vi "test_Multiple Local Enumerated Channel Command-Response Messages using Trigger with Padding and Protection.vi"(8 "error in (no error)":errorcluster, 11 "TestCase in":refnum<class "Common System Tests.lvclass">) -> (0 "error out":errorcluster, 3 "TestCase out":refnum<class "Common System Tests.lvclass">)   [LabVIEW 2018, in "Common System Tests.lvclass"]
uses:
  Common System Tests.lvclass
  C:/Dev/niveristand-custom-device-testing-tools/VeriStandTestCase/VeriStandTestCase.lvclass
  <vilib>/NI Veristand/Execution/Workspace/NI VeriStand - Set Multiple Channel Values.vi
  <vilib>/NI Veristand/Execution/Workspace/NI VeriStand - Get Multiple Channel Values.vi
  <vilib>/addons/_JKI Toolkits/VI Tester/TestCase.llb/TestCase.lvclass
  <vilib>/NI Veristand/Execution/Workspace/NI_VS Workspace ExecutionAPI.lvlib
  C:/Program Files (x86)/National Instruments/LabVIEW 2018/vi.lib/addons/_JKI Toolkits/VI Tester/TestCase.llb/TestCase.lvclass
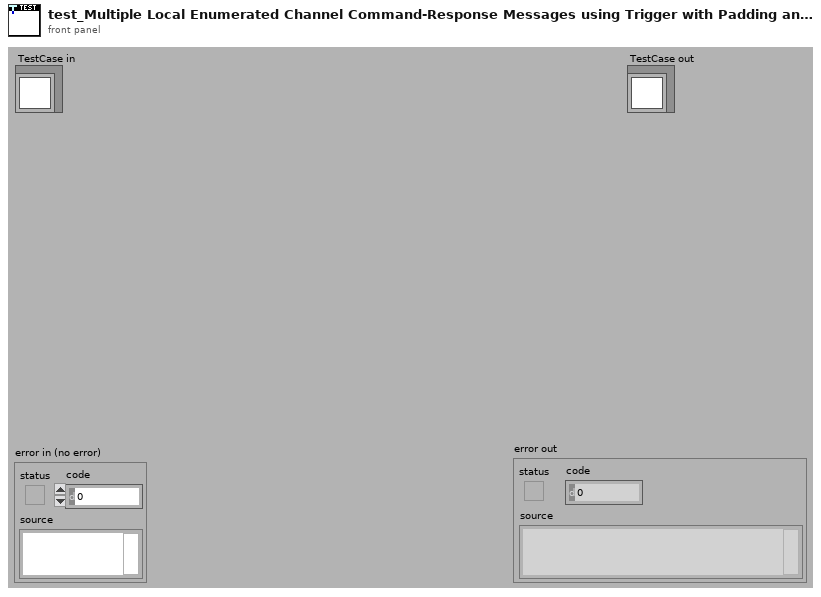
[diagram p1: front panel]
types:
  T1 = typedef "NI_VS Workspace ExecutionAPI.lvlib/WorkspaceAPI.ctl" = refnum<k24>
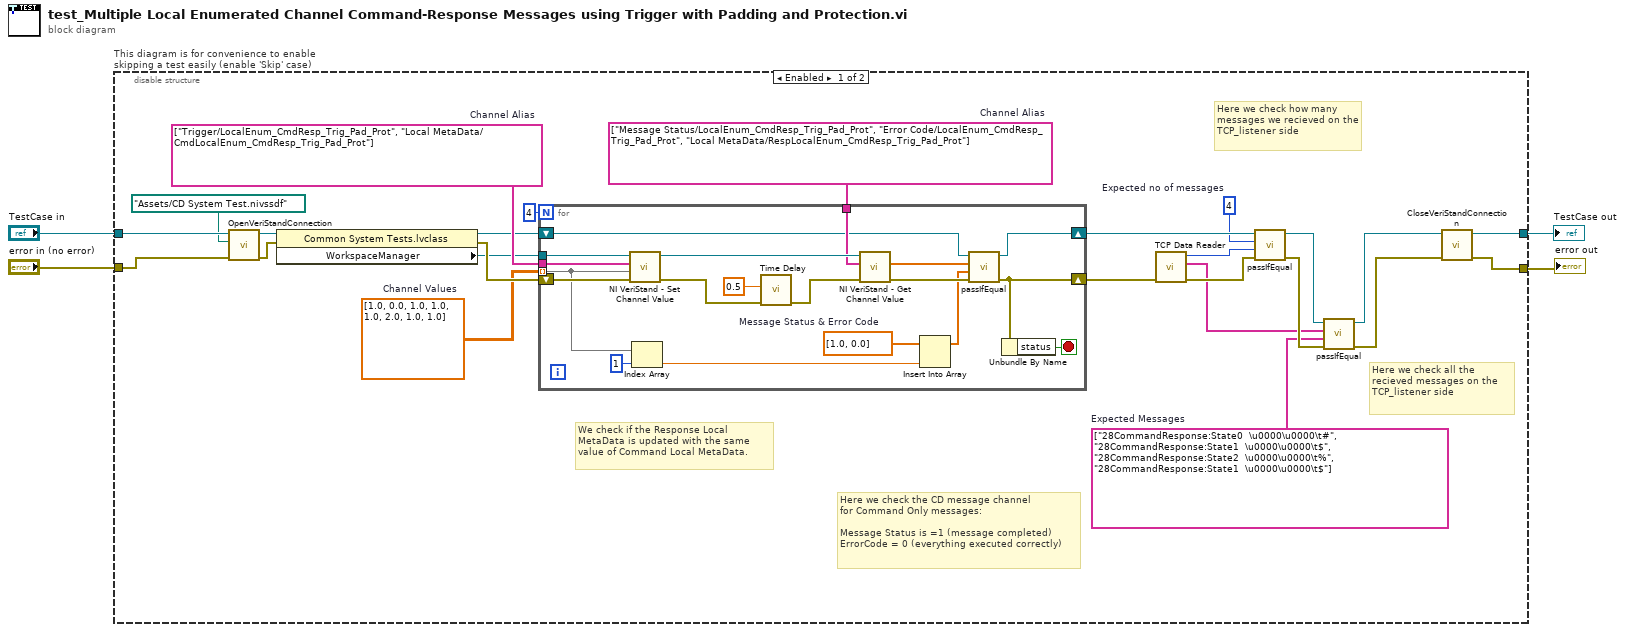
[diagram p0: block diagram]
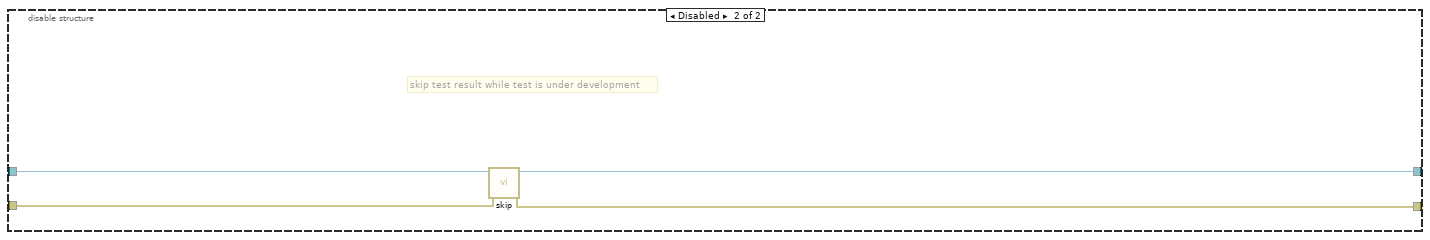
[diagram p2: hidden frame]
diagram:
  n1 = disable-structure "This diagram is for convenience to enable skipping a test easily (enable 'Skip' case)" shown="Enabled" {
    disable-tunnel: "TestCase in" -> [w27 w52]
    disable-tunnel: [w28 w50] -> w1
    disable-tunnel: [w29 w51] -> w3
    disable-tunnel: "error in (no error)" -> [w25 w49]
    frame Enabled {
      w5 = string[] ["28CommandResponse:State0  \u0000\u0000\t#", "28CommandResponse:State1  \u0000\u0000\t$", "28CommandResponse:State2  \u0000\u0000\t%", "28CommandResponse:State1  \u0000\u0000\t$"]  # Expected Messages
      w8 = 4  # Expected no of messages
      w17 = string[] ["Message Status/LocalEnum_CmdResp_Trig_Pad_Prot", "Error Code/LocalEnum_CmdResp_Trig_Pad_Prot", "Local MetaData/RespLocalEnum_CmdResp_Trig_Pad_Prot"]  # Channel Alias
      w20 = dbl[][] [[1.0, 0.0], [1.0, 1.0], [1.0, 2.0], [1.0, 1.0]]  # Channel Values
      w21 = string[] ["Trigger/LocalEnum_CmdResp_Trig_Pad_Prot", "Local MetaData/CmdLocalEnum_CmdResp_Trig_Pad_Prot"]  # Channel Alias
      # "We check if the Response Local MetaData is updated with the same value of Command Local MetaData."
      # "Here we check how many messages we recieved on the TCP_listener side"
      # "Here we check all the recieved messages on the TCP_listener side"
      # "Here we check the CD message channel\nfor Command Only messages:\n\nMessage Status is =1 (message completed)\nErrorCode = 0 (everything executed correctly)"
      n2 = call-dynamic "OpenVeriStandConnection.vi"("error in (no error)"=w25, "System Definition File"=path "Assets/CD System Test.nivssdf", "VeriStand Test Case in"=w27) -> ("error out"=w24:errorcluster, "VeriStand Test Case out"=w26:refnum<class "Common System Tests.lvclass">)  [unwired: 6 in, 1 out]
      n3 = property class="Common System Tests.lvclass"(reference=w26, error in=w24) -> (reference out=w18:refnum<class "Common System Tests.lvclass">, error out=w22:errorcluster, "WorkspaceManager"=w16:T1)
      n4 = for {
        N: 4 -> [_]
        tunnel: w16 -> [w48]
        tunnel: w21 -> [w46]
        tunnel: w20 -> [w33] mode=indexing
        shift-right: [w35] -> w7
        shift-left: w22 -> [w47]
        tunnel: w17 -> [w44]
        shift-right: [w39] -> w15
        shift-left: w18 -> [w40]
        stop <- w34 stop-if-true
        w36 = dbl[] [1.0, 0.0]  # Message Status & Error Code
        n5 = call-poly <vilib>:"NI VeriStand - Set Channel Value.vi"("error in (no error)"=w47, "Values"=w33, "Channels"=w46, "WorkspaceManager in"=w48) -> ("error out"=w42:errorcluster, "WorkspaceManager out"=w45:T1)  [unwired: 6 in]
        n6 = Index Array(array=w33, index=1) -> (element=w30:dbl)
        n7 = call "Time Delay"("error in (no error)"=w42, "Delay Time (s)"=0.5) -> ("error out"=w41:errorcluster)  [unwired: 9 in]
        n8 = call-poly <vilib>:"NI VeriStand - Get Channel Value.vi"("error in (no error)"=w41, "Channels"=w44, "WorkspaceManager in"=w45) -> ("error out"=w38:errorcluster, "Values"=w37:dbl[])  [unwired: 6 in, 1 out]
        n9 = Insert Into Array(array=w36, new element=w30) -> (w32:dbl[])  [unwired: 1 in]
        n10 = call-dynamic "passIfEqual.vi"("error in (no error)"=w38, "y"=w32, "x"=w37, "TestCase in"=w40) -> ("error out"=w35:errorcluster, "TestCase out"=w39:refnum<class "Common System Tests.lvclass">)  [unwired: 6 in]
        n11 = Unbundle By Name(w35) -> ("status"=w34:bool)
      }
      n12 = call "TCP Data Reader.vi"("error in (no error)"=w7) -> ("error out"=w13:errorcluster, "Recieved Messages"=w6:string[], "No of messages"=w9:i32)  [unwired: 8 in]
      n13 = call-dynamic "passIfEqual.vi"("error in (no error)"=w13, "y"=w9, "x"=w8, "TestCase in"=w15) -> ("error out"=w11:errorcluster, "TestCase out"=w14:refnum<class "Common System Tests.lvclass">)  [unwired: 6 in]
      n14 = call-dynamic "passIfEqual.vi"("error in (no error)"=w11, "y"=w5, "x"=w6, "TestCase in"=w14) -> ("error out"=w10:errorcluster, "TestCase out"=w12:refnum<class "Common System Tests.lvclass">)  [unwired: 6 in]
      n15 = call-dynamic "CloseVeriStandConnection.vi"("error in (no error)"=w10, "VeriStand Test Case in"=w12) -> ("error out"=w29:errorcluster, "VeriStand Test Case out"=w28:refnum<class "Common System Tests.lvclass">)  [unwired: 8 in]
    }
    frame Disabled {
      # "skip test result while test is under development"
      n16 = call <vilib>:"skip.vi"("error in (no error)"=w49, "TestCase in"=w52) -> ("error out"=w51:errorcluster, "TestCase out"=w50:refnum<class "Common System Tests.lvclass">)  [unwired: 8 in]
    }
  }
  "error out" <- w3
  "TestCase out" <- w1
